vi "Write Modulation.vi"(8 "error in (no error)":errorcluster, 10 "Modulation":T1, 11 "Change Laser Modulation in":refnum<class "Change Laser Modulation.lvclass">) -> (0 "error out":errorcluster, 3 "Change Laser Modulation out":refnum<class "Change Laser Modulation.lvclass">)   [LabVIEW 2014, in "Change Laser Modulation.lvclass"]
uses:
  Change Laser Modulation.lvclass
  reusable/PAS/Controls/Modulation Type.ctl
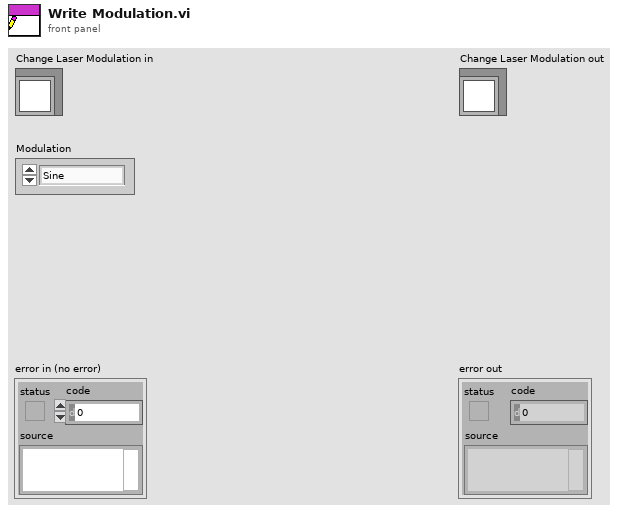
[diagram p1: front panel]
types:
  T1 = typedef "Modulation Type.ctl" = enum16{"Sine", "Square"}
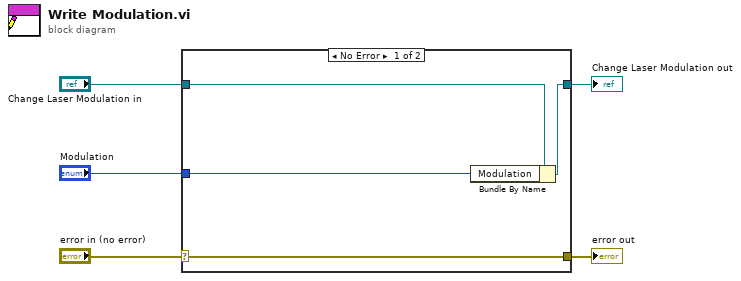
[diagram p0: block diagram]
diagram:
  n1 = case shown="No Error" "error in (no error)" {
    selector: "error in (no error)" -> [w9 w10]
    tunnel: [w9 w10] -> w4
    tunnel: [w7 w11] -> w2
    tunnel: "Change Laser Modulation in" -> [w8 w11]
    tunnel: "Modulation" -> [w6 _]
    frame No Error {
      n2 = Bundle By Name(cluster=w8, "Modulation"=w6) -> (w7:refnum<class "Change Laser Modulation.lvclass">)
    }
    frame Error {
    }
  }
  "error out" <- w4
  "Change Laser Modulation out" <- w2
